vi "Example Graph.vi"() -> ()   [LabVIEW 2010]
uses:
  C:/tf/play/labview/Tinkerforge.dll
  Tinkerforge.dll
panel:
  in  "stop":bool
  out "graph":sgl[](graph)
  in  "uid":string="amb"
  in  "port":i32=4223
  in  "host":string="localhost"
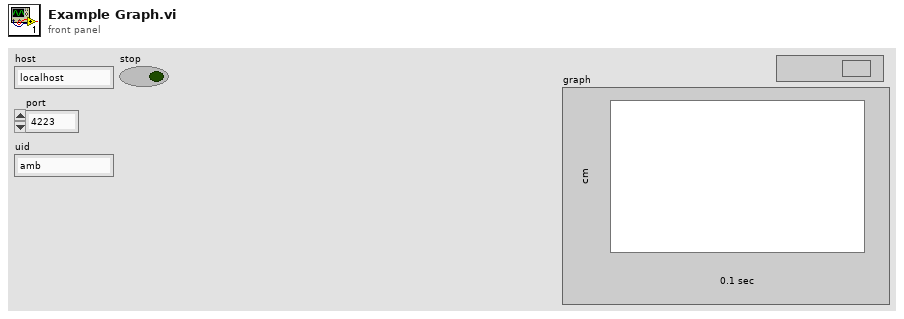
[diagram p1: front panel]
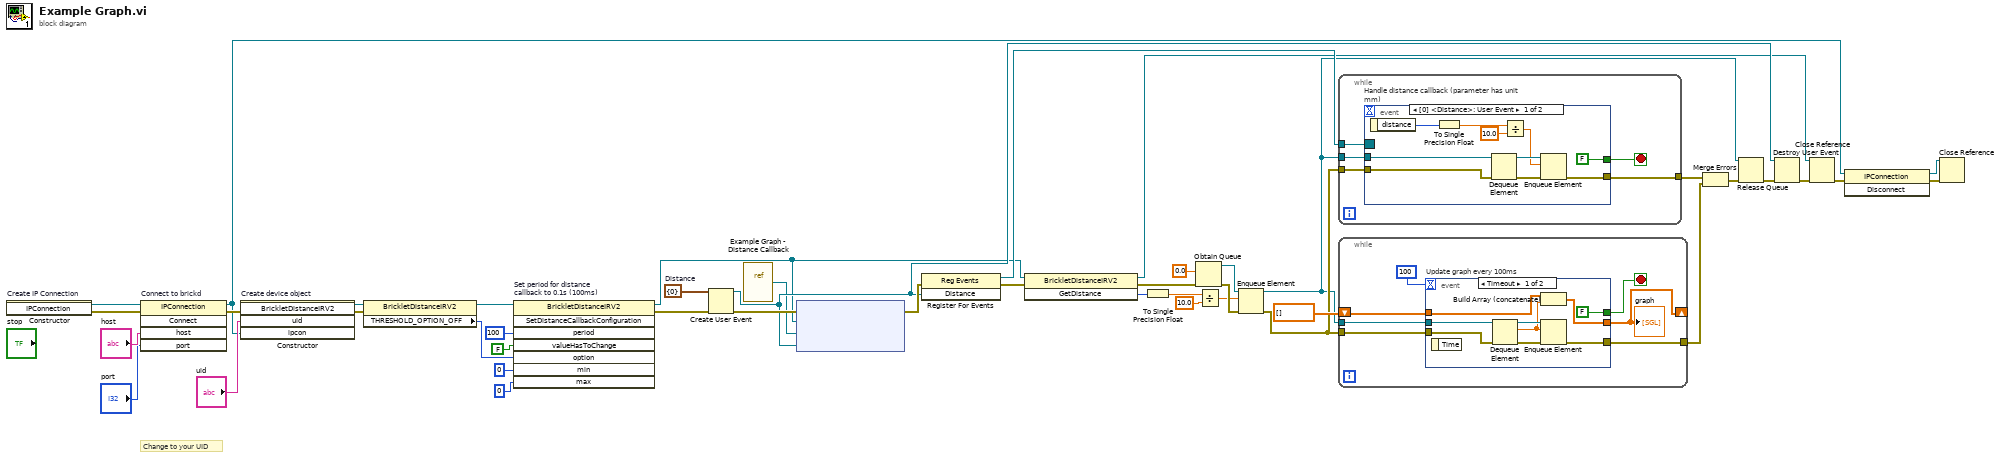
[diagram p0: block diagram]
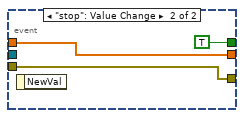
[diagram p2: hidden frame]
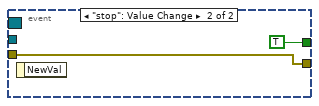
[diagram p3: hidden frame]
diagram:
  w30 = cluster{"distance":i32} {"distance"=0}  # Distance
  # "Change to your UID"
  n1 = constructor on="Create IP Connection" class="IPConnection"() -> (reference out=w44:refnum<k24>, error out=w17:errorcluster)  [unwired: 3 in, 1 out]
  n2 = invoke on="Connect to brickd" class="IPConnection" method="Connect"(reference=w44, error in=w17, "host"="host", "port"="port") -> (reference out=w37:refnum<k24>, error out=w40:errorcluster)  [unwired: 1 in, 3 out]
  n3 = constructor on="Create device object" class="BrickletDistanceIRV2"(error in=w40, "uid"="uid", "ipcon"=w37) -> (reference out=w4:refnum<k24>, error out=w5:errorcluster)  [unwired: 2 in, 3 out]
  n4 = property class="BrickletDistanceIRV2"(reference=w4, error in=w5) -> (reference out=w3:refnum<k24>, "THRESHOLD_OPTION_OFF"=w2:u16)  [unwired: 1 out]
  n5 = invoke on="Set period for distance\ncallback to 0.1s (100ms)" class="BrickletDistanceIRV2" method="SetDistanceCallbackConfiguration"(reference=w3, "period"=i64 100, "valueHasToChange"=FALSE, "option"=w2, "min"=0, "max"=0) -> (reference out=w16:refnum<k24>, error out=w29:errorcluster)  [unwired: 2 in, 6 out]
  n6 = Create User Event(user event datatype=w30, error in=w29) -> (user event=w32:refnum<user-event>, error out=w35:errorcluster)
  n7 = vi-ref "Example Graph - Distance Callback.vi"() -> ("vi reference"=w1:refnum<vi>)
  n8 = node ("Register Event Callback")(w35, w16, w1, w32) -> (w34:errorcluster)  [unwired: 1 in, 1 out]
  n9 = register-events(error in=w34, w32) -> (reference out=w33:refnum<event-registration>, error out=w14:errorcluster)  [unwired: 1 in]
  n10 = invoke class="BrickletDistanceIRV2" method="GetDistance"(reference=w16, error in=w14) -> (reference out=w15:refnum<k24>, error out=w13:errorcluster, "GetDistance"=w9:i32)  [unwired: 1 in]
  n11 = To Single Precision Float(number=w9) -> (single precision float=w12:sgl)
  n12 = Obtain Queue(element data type=sgl 0.0, error in (no error)=w13) -> (queue out=w21:refnum<queue>, error out=w23:errorcluster)  [unwired: 3 in, 1 out]
  n13 = Divide(x=w12, y=sgl 10.0) -> (x/y=w10:sgl)
  n14 = Enqueue Element(queue=w21, element=w10, error in (no error)=w23) -> (queue out=w18:refnum<queue>, error out=w22:errorcluster)  [unwired: 1 in, 1 out]
  n15 = while {
    tunnel: w33 -> [w49]
    tunnel: [w47] -> w26
    tunnel: w22 -> [w48]
    tunnel: w18 -> [w46]
    stop <- w45 stop-if-true
    n16 = event "Handle distance callback (parameter has unit mm)" shown="[0] <Distance>: User Event" {
      selector: w49 -> [_ _]
      dyn-events: _ -> [_ _]
      timeout: _ -> [_ _]
      tunnel: w48 -> [w56 w60]
      tunnel: [w54 w60] -> w47
      tunnel: w46 -> [w53 _]
      tunnel: [FALSE TRUE] -> w45
      event User Event {
        n17 = event-data() -> ("distance"=w57:i32)  [unwired: 1 in]
        n18 = To Single Precision Float(number=w57) -> (single precision float=w58:sgl)
        n19 = Dequeue Element(queue=w53, error in (no error)=w56) -> (queue out=w52:refnum<queue>, error out=w55:errorcluster)  [unwired: 1 in, 2 out]
        n20 = Divide(x=w58, y=sgl 10.0) -> (x/y=w51:sgl)
        n21 = Enqueue Element(queue=w52, element=w51, error in (no error)=w55) -> (error out=w54:errorcluster)  [unwired: 1 in, 2 out]
      }
      event "stop": Value Change {
        n22 = event-data() -> ()  [unwired: 1 in, 1 out]
      }
    }
  }
  n23 = while {
    tunnel: [w64] -> w27
    tunnel: w22 -> [w65]
    shift-right: [w66] -> _
    shift-left: sgl[] [] -> [w67]
    tunnel: w18 -> [w63]
    stop <- w62 stop-if-true
    n24 = event "Update graph every 100ms" shown="[0] Timeout" {
      selector: _ -> [_ _]
      dyn-events: _ -> [_ _]
      timeout: 100 -> [_ _]
      tunnel: [w77 w79] -> w66
      tunnel: w67 -> [w70 w79]
      tunnel: w65 -> [w76 w78]
      tunnel: [w73 w78] -> w64
      tunnel: w63 -> [w75 _]
      tunnel: [FALSE TRUE] -> w62
      event Timeout {
        n25 = event-data() -> ()  [unwired: 1 in, 1 out]
        n26 = Dequeue Element(queue=w75, error in (no error)=w76) -> (queue out=w72:refnum<queue>, element=w71:sgl, error out=w74:errorcluster)  [unwired: 1 in, 1 out]
        n27 = Build Array (concatenate)(w70, w71) -> (w77:sgl[])
        n28 = Enqueue Element(queue=w72, element=w71, error in (no error)=w74) -> (error out=w73:errorcluster)  [unwired: 1 in, 2 out]
      }
      event "stop": Value Change {
        n29 = event-data() -> ()  [unwired: 1 in, 1 out]
      }
    }
    "graph" <- w66
  }
  n30 = Merge Errors(w26, w27) -> (w20:errorcluster)
  n31 = Release Queue(queue=w18, error in (no error)=w20) -> (error out=w19:errorcluster)  [unwired: 1 in, 2 out]
  n32 = Destroy User Event(user event=w32, error in=w19) -> (error out=w31:errorcluster)
  n33 = Close Reference(reference=w15, error in (no error)=w31) -> (error out=w39:errorcluster)
  n34 = invoke class="IPConnection" method="Disconnect"(reference=w37, error in=w39) -> (reference out=w36:refnum<k24>, error out=w38:errorcluster)  [unwired: 1 in, 1 out]
  n35 = Close Reference(reference=w36, error in (no error)=w38) -> ()  [unwired: 1 out]
